vi "LSCI332WriteCalib.vi"(0 "VISA Rsrc":refnum<visa-resource-name>="GPIB0::12::INSTR" caption="Adresse du contrôlleur", 1 "Nom":string="CourbeTest", 2 "No de série":string="Standard", 5 "ValCalib":dbl[][](array[numeric]) caption="Valeurs de Calibration", 7 "No Courbe":u32=21 min=21 max=41 step=1, 9 "Coefficient":u16(ring)=2 items=["Faites un choix", "négatif", "positif"], 11 "error in":errorcluster, 12 "Format":u16(ring)=2 items=["Faites un choix", "mV/K", "V/K", "Ohm/K", "log Ohm/K"], 13 "TLim":dbl=475.0 caption="T° de Contrôle Max (K)") -> (4 "Complété":bool caption="Écriture Complété", 6 "Nom Out":string="CourbeTest", 8 "No de série Out":string="Standard", 15 "error out":errorcluster)   [LabVIEW 2019]
doc: "Ce Vi écrit l'entête et les points d'une courbe de calibration dans l'emplacement spécifié du contrôlleur de température"
uses:
  <vilib>/Utility/error.llb/DialogType.ctl
panel:
  # "Sortie Capteur"
  # "Température (K)"
  # "+5"
  # "+10"
  # "+15"
  # "+20"
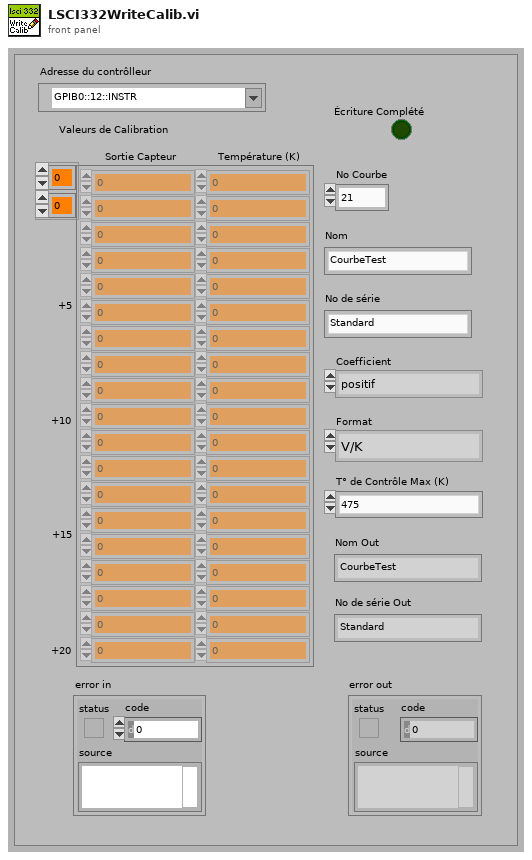
[diagram p1: front panel]
types:
  T1 = enum16{"Vérif Données", "Écrit Entête", "Écrit Points", "Erreur"}
  T2 = typedef "DialogType.ctl" = u16
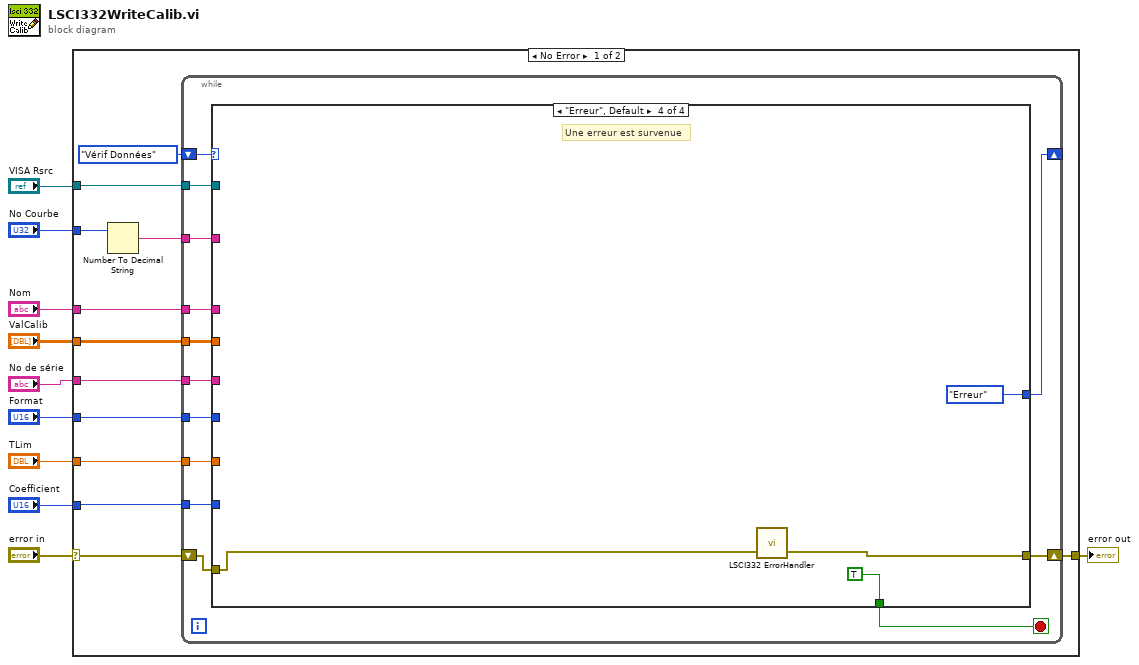
[diagram p0: block diagram]
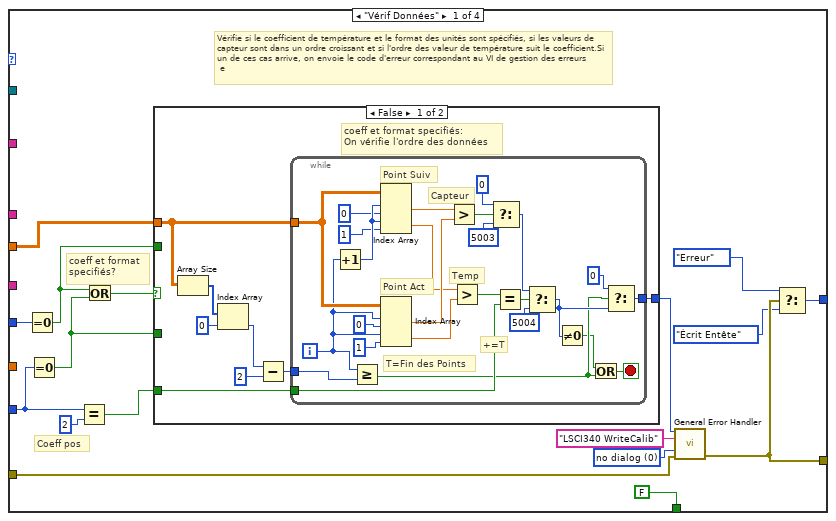
[diagram p2: hidden frame]
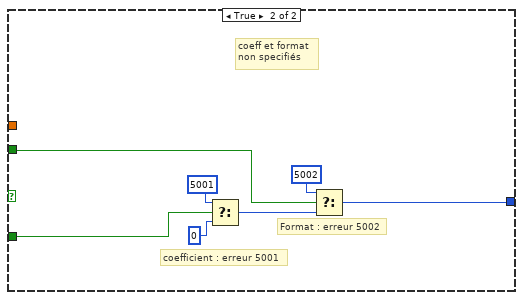
[diagram p3: hidden frame]
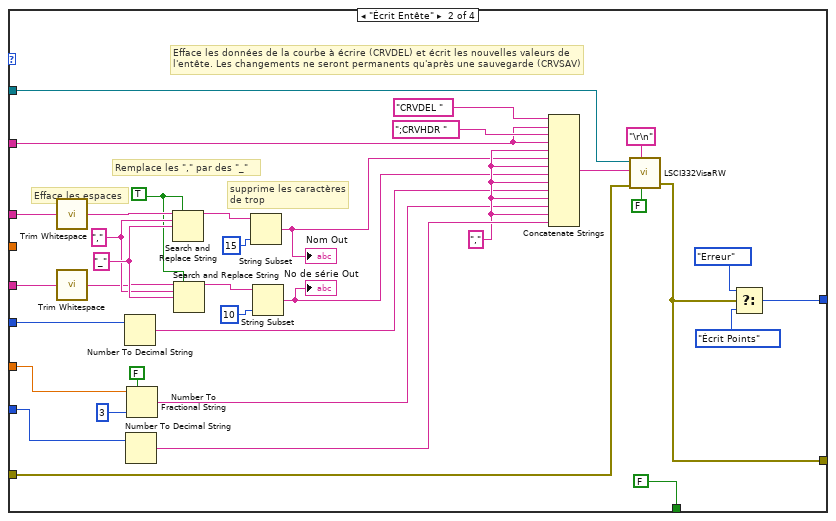
[diagram p4: hidden frame]
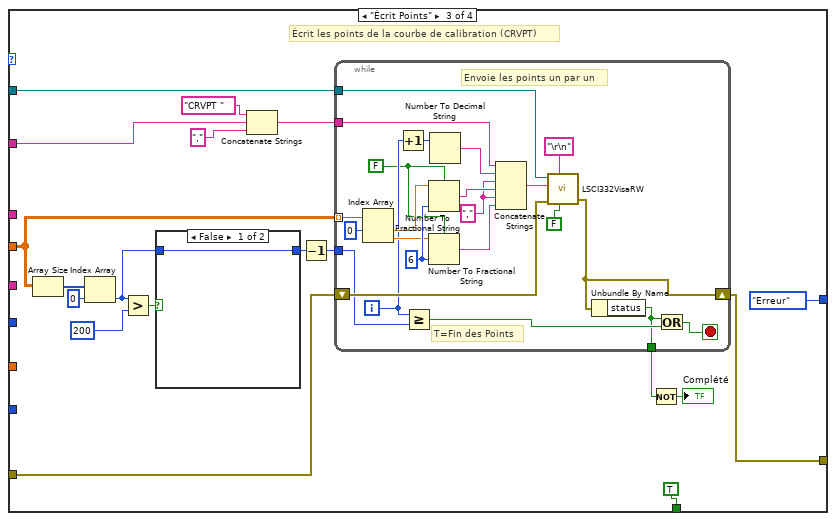
[diagram p5: hidden frame]
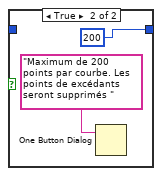
[diagram p6: hidden frame]
diagram:
  n1 = case shown="No Error" "error in" {
    selector: "error in" -> [w20 w178]
    tunnel: "VISA Rsrc" -> [w13 _]
    tunnel: "ValCalib" -> [w19 _]
    tunnel: "Coefficient" -> [w22 _]
    tunnel: "Format" -> [w21 _]
    tunnel: "Nom" -> [w18 _]
    tunnel: "No de série" -> [w17 _]
    tunnel: "TLim" -> [w16 _]
    tunnel: "No Courbe" -> [w15 _]
    tunnel: [w12 w178] -> w1
    frame No Error {
      n2 = Number To Decimal String(number=w15) -> (decimal integer string=w14:string)  [unwired: 1 in]
      n3 = while {
        tunnel: w22 -> [w35]
        tunnel: w21 -> [w34]
        shift-right: [w33] -> w12
        shift-left: w20 -> [w31]
        tunnel: w19 -> [w32]
        tunnel: w18 -> [w29]
        tunnel: w17 -> [w28]
        tunnel: w16 -> [w27]
        tunnel: w14 -> [w26]
        tunnel: w13 -> [w25]
        shift-right: [w23] -> _
        shift-left: T1."Vérif Données" -> [w24]
        stop <- w30 stop-if-true
        n4 = case shown="\"Erreur\", Default" w24 {
          tunnel: w35 -> [w50 w107 _ _]
          tunnel: w34 -> [w51 w109 _ _]
          tunnel: w31 -> [w48 w100 w138 w177]
          tunnel: [w39 w99 w133 w176] -> w33
          tunnel: w32 -> [w46 _ w139 _]
          tunnel: [FALSE FALSE TRUE TRUE] -> w30
          tunnel: w29 -> [_ w111 _ _]
          tunnel: w28 -> [_ w110 _ _]
          tunnel: w27 -> [_ w108 _ _]
          tunnel: w26 -> [_ w106 w140 _]
          tunnel: w25 -> [_ w103 w145 _]
          tunnel: [w36 w96 T1."Erreur" T1."Erreur"] -> w23
          frame "Vérif Données" {
            w49 = T2 0 items=["no dialog", "OK message", "continue or stop message", "OK message + warnings", "continue/stop + warnings"] ("type of dialog (OK msg:1)")
            # "coeff et format\nspecifiés?"
            # "Vérifie si le coefficient de température et le format des unités sont spécifiés, si les valeurs de capteur sont dans un ordre croissant et si l'ordre des valeur de température suit le coefficient.Si un de ces cas arrive, on envoie le code d'erreur correspondant au VI de gestion des erreurs\n e"
            # "Coeff pos"
            n5 = Equal To 0?(x=w51) -> (x = 0?=w43:bool)
            n6 = Equal To 0?(x=w50) -> (x = 0?=w44:bool)
            n7 = Equal?(x=w50, y=u16 2) -> (x = y?=w41:bool)
            n8 = Or(x=w43, y=w44) -> (x .or. y?=w45:bool)
            n9 = case shown="False" w45 {
              tunnel: w46 -> [w59 _]
              tunnel: w41 -> [w57 _]
              tunnel: w44 -> [_ w88]
              tunnel: w43 -> [_ w89]
              tunnel: [w60 w87] -> w42
              frame False {
                # "coeff et format specifiés:\nOn vérifie l'ordre des données"
                n10 = Array Size(array=w59) -> (size(s)=w58:i32[])
                n11 = Index Array(array=w58, index=0) -> (element=w54:i32)
                n12 = Subtract(x=w54, y=2) -> (x-y=w55:i32)
                n13 = while {
                  tunnel: w59 -> [w69]
                  tunnel: w57 -> [w77]
                  tunnel: [w66] -> w60
                  tunnel: w55 -> [w67]
                  i -> [w68]
                  stop <- w63 stop-if-true
                  # "T=Fin des Points"
                  # "+=T"
                  # "Temp"
                  # "Capteur"
                  # "Point Suiv"
                  # "Point Act"
                  n14 = Increment(x=w68) -> (x+1=w86:i32)
                  n15 = Greater Or Equal?(x=w68, y=w67) -> (x >= y?=w62:bool)
                  n16 = Index Array(array=w69, index (row) #1=w86, index (col) #1=0 ("disabled index (col)"), index (row) #2=w86, index (col) #2=1 ("disabled index (col)")) -> (element #1=w82:dbl, element #2=w80:dbl)
                  n17 = Index Array(array=w69, index (row) #1=w68, index (col) #1=0 ("disabled index (col)"), index (row) #2=w68, index (col) #2=1 ("disabled index (col)")) -> (element #1=w81:dbl, element #2=w79:dbl)
                  n18 = Greater?(x=w82, y=w81) -> (0:w76:bool)
                  n19 = Greater?(x=w80, y=w79) -> (0:w78:bool)
                  n20 = Select(t=0, s=w76, f=5003) -> (s? t:f=w70:i32)
                  n21 = Equal?(x=w78, y=w77) -> (x = y?=w71:bool)
                  n22 = Select(t=w70, s=w71, f=5004) -> (s? t:f=w65:i32)
                  n23 = Not Equal To 0?(x=w65) -> (x != 0?=w61:bool)
                  n24 = Or(x=w61, y=w62) -> (x .or. y?=w63:bool)
                  n25 = Select(t=0, s=w62, f=w65) -> (s? t:f=w66:i32)
                }
              }
              frame True {
                # "Format : erreur 5002"
                # "coefficient : erreur 5001"
                # "coeff et format\nnon specifiés"
                n26 = Select(t=5001, s=w88, f=0) -> (s? t:f=w93:i32)
                n27 = Select(t=5002, s=w89, f=w93) -> (s? t:f=w87:i32)
              }
            }
            n28 = call <vilib>:"General Error Handler.vi"("[error code] (0)"=w42, "[error source] (\" \")"="LSCI340 WriteCalib" ("[error source] (\" \")"), "type of dialog (OK msg:1)"=w49, "error in (no error)"=w48) -> ("error out"=w39:errorcluster)  [unwired: 7 in, 4 out]
            n29 = Select(t=T1."Erreur", s=w39, f=T1."Écrit Entête") -> (s? t:f=w36:T1)
          }
          frame "Écrit Entête" {
            w124 = ","
            w105 = TRUE
            w115 = "_"
            w114 = ","
            # "Efface les données de la courbe à écrire (CRVDEL) et écrit les nouvelles valeurs de l'entête. Les changements ne seront permanents qu'après une sauvegarde (CRVSAV)"
            # "supprime les caractères de trop"
            # "Remplace les \",\" par des \"_\""
            # "Efface les espaces"
            n30 = call <vilib>:"Trim Whitespace.vi"("string"=w111) -> ("trimmed string"=w112:string)  [unwired: 1 in]
            n31 = call <vilib>:"Trim Whitespace.vi"("string"=w110) -> ("trimmed string"=w113:string)  [unwired: 1 in]
            n32 = Number To Decimal String(number=w109) -> (decimal integer string=w121:string)  [unwired: 1 in]
            n33 = Number To Decimal String(number=w107) -> (decimal integer string=w125:string)  [unwired: 1 in]
            n34 = Number To Fractional String(use system decimal point (T)=FALSE, number=w108, precision (6)=3) -> (F-format string=w123:string)  [unwired: 1 in]
            n35 = Search and Replace String(replace all?=w105, input string=w112, search string=w114, replace string=w115) -> (result string=w116:string)  [unwired: 4 in, 3 out]
            n36 = Search and Replace String(replace all?=w105, input string=w113, search string=w114, replace string=w115) -> (result string=w118:string)  [unwired: 4 in, 3 out]
            n37 = String Subset(string=w116, length (rest)=15) -> (substring=w95:string)  [unwired: 1 in]
            "Nom Out" <- w95
            n38 = String Subset(string=w118, length (rest)=10) -> (substring=w94:string)  [unwired: 1 in]
            "No de série Out" <- w94
            n39 = Concatenate Strings("CRVDEL ", w106, ";CRVHDR ", w106, w124, w95, w124, w94, w124, w121, w124, w123, w124, w125) -> (w104:string)
            n40 = call <userlib>:"LSCI332VisaRW.vi"("Lecture?(T)"=FALSE, "error in (no error)"=w100, "EOS (Aucun)"="\r\n", "ChaineCom"=w104, "VISA Rsrc"=w103) -> ("error out"=w99:errorcluster)  [unwired: 2 in, 3 out]
            n41 = Select(t=T1."Erreur", s=w99, f=T1."Écrit Points") -> (s? t:f=w96:T1)
          }
          frame "Écrit Points" {
            # "Écrit les points de la courbe de calibration (CRVPT)"
            n42 = Array Size(array=w139) -> (size(s)=w144:i32[])
            n43 = Index Array(array=w144, index=0) -> (element=w137:i32)
            n44 = Greater?(x=w137, y=200) -> (0:w141:bool)
            n45 = case shown="False" w141 {
              tunnel: [w171 200] -> w136
              tunnel: w137 -> [w171 _]
              frame False {
              }
              frame True {
                n46 = One Button Dialog(message="Maximum de 200 points par courbe. Les points de excédants seront supprimés ") -> ()  [unwired: 1 in, 1 out]
              }
            }
            n47 = Concatenate Strings("CRVPT ", w140, ",") -> (w135:string)
            n48 = Decrement(x=w136) -> (x-1=w134:i32)
            n49 = while {
              tunnel: w145 -> [w170]
              tunnel: w139 -> [w166] mode=indexing
              shift-right: [w164] -> w133
              shift-left: w138 -> [w167]
              tunnel: w134 -> [w163]
              tunnel: w135 -> [w150]
              tunnel: [w149] -> w130
              i -> [w157]
              stop <- w162 stop-if-true
              w148 = FALSE ("use system decimal point (T)")
              w161 = 6
              w151 = ","
              # "Envoie les points un par un"
              # "T=Fin des Points"
              n50 = Index Array(array=w166, index #1=0 ("index")) -> (element #1=w160:dbl, element #2=w159:dbl)  [unwired: 1 in]
              n51 = Increment(x=w157) -> (x+1=w158:i32)
              n52 = Greater Or Equal?(x=w157, y=w163) -> (x >= y?=w156:bool)
              n53 = Number To Fractional String(use system decimal point (T)=w148, number=w160, precision (6)=w161) -> (F-format string=w153:string)  [unwired: 1 in]
              n54 = Number To Fractional String(use system decimal point (T)=w148, number=w159, precision (6)=w161) -> (F-format string=w152:string)  [unwired: 1 in]
              n55 = Number To Decimal String(number=w158) -> (decimal integer string=w154:string)  [unwired: 1 in]
              n56 = Concatenate Strings(w150, w154, w151, w153, w151, w152) -> (w155:string)
              n57 = call <userlib>:"LSCI332VisaRW.vi"("Lecture?(T)"=FALSE, "error in (no error)"=w167, "EOS (Aucun)"="\r\n", "ChaineCom"=w155, "VISA Rsrc"=w170) -> ("error out"=w164:errorcluster)  [unwired: 2 in, 3 out]
              n58 = Unbundle By Name(w164) -> ("status"=w149:bool)
              n59 = Or(x=w149, y=w156) -> (x .or. y?=w162:bool)
            }
            n60 = Not(x=w130) -> (.not. x?=→"Complété":bool)
          }
          frame "Erreur", Default {
            # "Une erreur est survenue"
            n61 = call <userlib>:"LSCI332 ErrorHandler.vi"("error in (no error)"=w177) -> ("error out"=w176:errorcluster)  [unwired: 1 in, 1 out]
          }
        }
      }
    }
    frame Error {
    }
  }
  "error out" <- w1
